vi "Configure Channel.vi"(8 "error in (no error)":errorcluster, 9 "Config Channel":T1={"Channel (0: Channel 1)"=0, "Vertical Coupling (1: DC)"=1, "Probe Attenuation (10: 10X)"=10, "Vertical Range (10.0 V/div)"=10.0, "Vertical Offset (0.0 divs)"=0.0, "Bandwidth (0: MAX Bandwidth)"=0, "Enable Channel (True)"=TRUE} {"Bandwidth (0: MAX Bandwidth)" items=["MAX Bandwidth", "Unlimited"]; "Probe Attenuation (10: 10X)" items=["1"=1, "10"=10, "20"=20, "50"=50, "100"=100, "500"=500, "1000"=1000]; "Vertical Coupling (1: DC)" items=["AC", "DC", "Ground"]; "Channel (0: Channel 1)" items=["Channel 1", "Channel 2", "Channel 3", "Channel 4", "Math", "Reference A", "Reference B", "Reference C", "Reference D"]}, 11 "Tektronic in":refnum<class "Tektronic.lvclass">) -> (0 "error out":errorcluster, 3 "Tektronic out":refnum<class "Tektronic.lvclass">)   [LabVIEW 2020, in "Controlador.lvlib" / "Tektronic.lvclass"]
uses:
  Tektronic/Tektronic.lvclass
  Tektronic/Tektronic.lvclass/Tektronic.ctl
  <instrlib>/Tektronix TDS 200 1000 2000 Series/Tektronix TDS 200 1000 2000 Series.lvlib
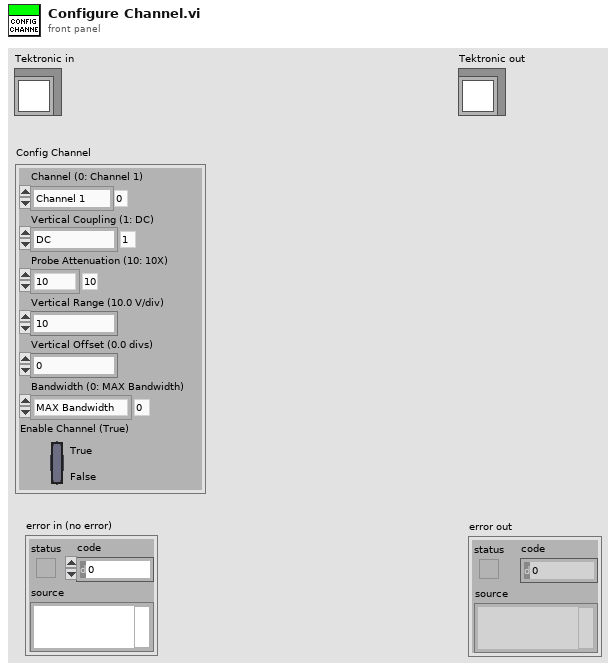
[diagram p1: front panel]
types:
  T1 = cluster{"Channel (0: Channel 1)":i32, "Vertical Coupling (1: DC)":i32, "Probe Attenuation (10: 10X)":i32, "Vertical Range (10.0 V/div)":dbl, "Vertical Offset (0.0 divs)":dbl, "Bandwidth (0: MAX Bandwidth)":i32, "Enable Channel (True)":bool}
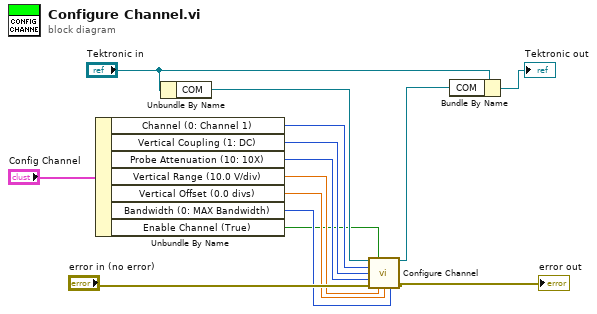
[diagram p0: block diagram]
diagram:
  n1 = Unbundle By Name("Config Channel") -> ("Channel (0: Channel 1)"=w7:i32, "Vertical Coupling (1: DC)"=w6:i32, "Probe Attenuation (10: 10X)"=w5:i32, "Vertical Range (10.0 V/div)"=w4:dbl, "Vertical Offset (0.0 divs)"=w3:dbl, "Bandwidth (0: MAX Bandwidth)"=w2:i32, "Enable Channel (True)"=w1:bool)
  n2 = Unbundle By Name("Tektronic in") -> ("COM"=w9:refnum<visa-resource-name>)
  n3 = call <instrlib>:"Configure Channel.vi"("VISA resource name"=w9, "Enable Channel (True)"=w1, "Channel (0: Channel 1)"=w7, "Vertical Coupling (1: DC)"=w6, "Probe Attenuation (10: 10X)"=w5, "error in (no error)"="error in (no error)", "Vertical Range (10.0 V/div)"=w4, "Vertical Offset (0.0 divs)"=w3, "Bandwidth (0: MAX Bandwidth)"=w2) -> ("VISA resource name out"=w10:refnum<visa-resource-name>, "error out"=→"error out":errorcluster)  [unwired: 5 in]
  n4 = Bundle By Name(cluster="Tektronic in", "COM"=w10) -> (→"Tektronic out":refnum<class "Tektronic.lvclass">)
